vi "test-VAttributes-Merge2.vi"(8 "error in (no error)":errorcluster, 11 "TestCase in":refnum<class "MyTestCase.lvclass">) -> (0 "error out":errorcluster, 3 "TestCase out":refnum<class "MyTestCase.lvclass">)   [LabVIEW 2019, in "MyTestCase.lvclass"]
uses:
  MyTestCase.lvclass
  <vilib>/addons/_JKI Toolkits/VI Tester/TestCase.llb/TestCase.lvclass
  C:/Program Files (x86)/National Instruments/LabVIEW 2019/vi.lib/addons/_JKI Toolkits/VI Tester/TestCase.llb/TestCase.lvclass
panel:
  out "VAttributes A after B->A 2":variant
  out "VAttributes A after B->A":variant
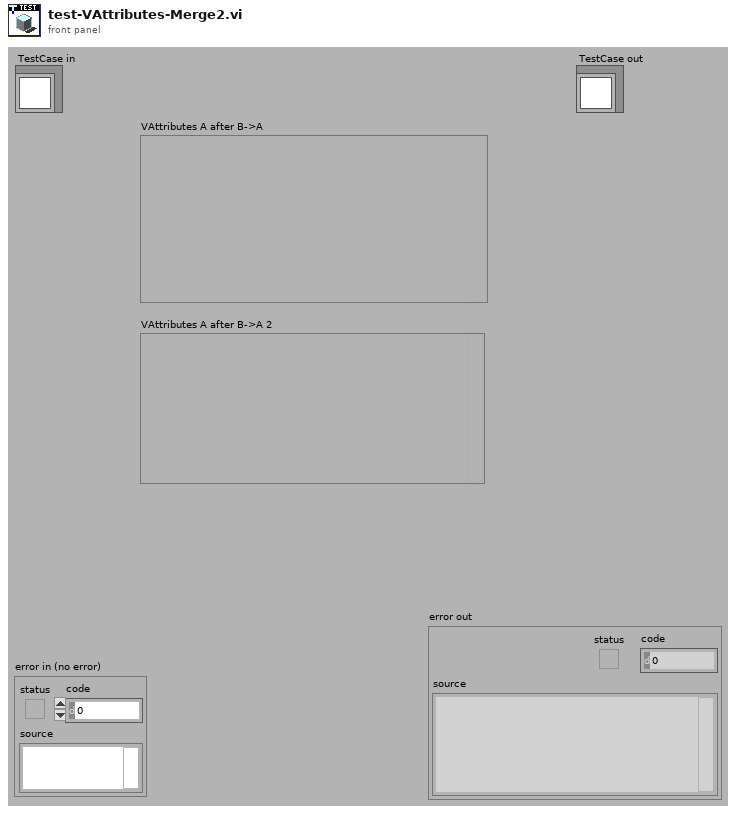
[diagram p1: front panel]
types:
  T1 = cluster{"bool":bool, "Cluster":cluster{"cluster":cluster{"cluster":cluster{"numeric":i32, "string":string}, "numeric":i32, "string":string}, "numeric":i32, "string":string}, "numeric":i32, "string":string, "string2":string}
  T2 = cluster{"numeric":i32, "string":string, "Cluster":cluster{"numeric":i32, "string":string, "cluster":cluster{"numeric":i32, "string":string, "cluster":cluster{"numeric":i32, "string":string}}}}
  T3 = cluster{"bool":bool, "string2":string, "cluster":cluster{"numeric":i32, "string":string, "cluster":cluster{"numeric":i32, "string":string}}}
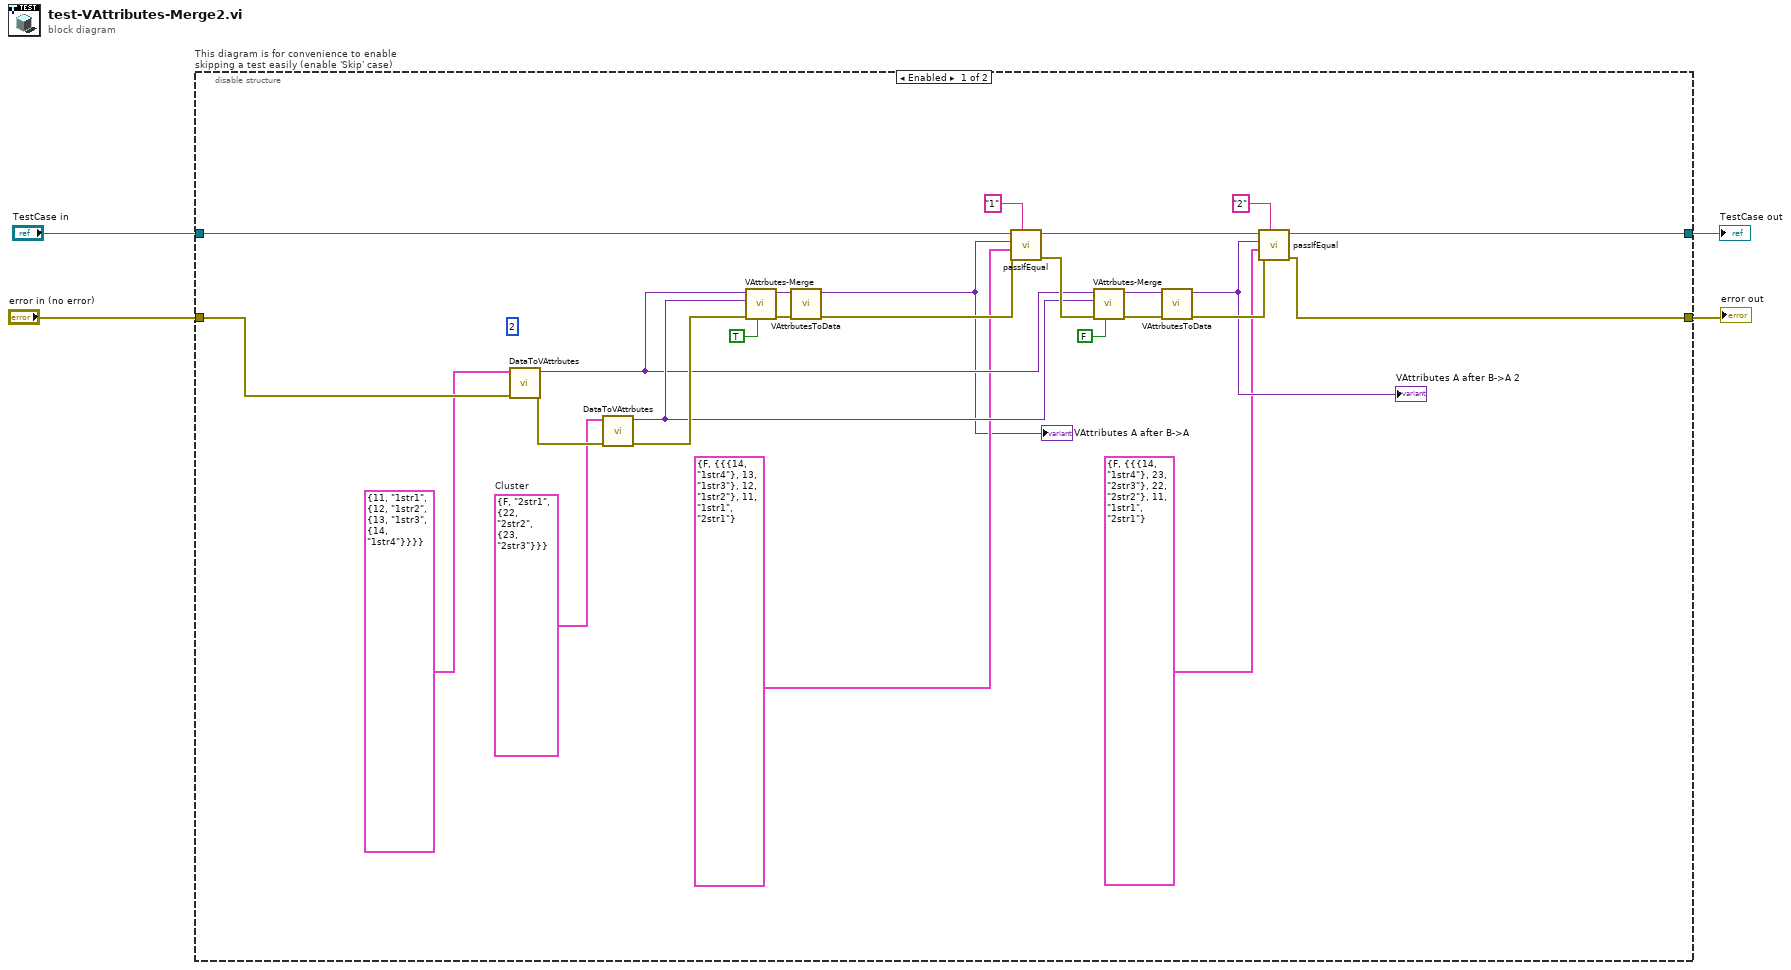
[diagram p0: block diagram]
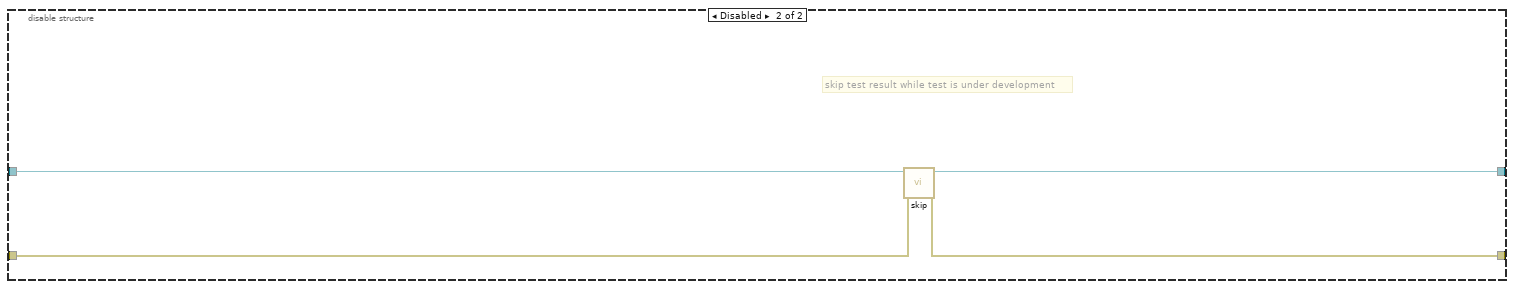
[diagram p2: hidden frame]
diagram:
  n1 = disable-structure "This diagram is for convenience to enable skipping a test easily (enable 'Skip' case)" shown="Enabled" {
    disable-tunnel: "TestCase in" -> [w27 w34]
    disable-tunnel: [w20 w32] -> w1
    disable-tunnel: [w18 w33] -> w3
    disable-tunnel: "error in (no error)" -> [w28 w31]
    frame Enabled {
      w16 = T3 {"bool"=FALSE, "string2"="2str1", "cluster"={"numeric"=22, "string"="2str2", "cluster"={"numeric"=23, "string"="2str3"}}}  # Cluster
      (unwired) 2
      n2 = call "DataToVAttrbutes.vi"("error in (no error)"=w28, "data"=T2 {"numeric"=11, "string"="1str1", "Cluster"={"numeric"=12, "string"="1str2", "cluster"={"numeric"=13, "string"="1str3", "cluster"={"numeric"=14, "string"="1str4"}}}} ("Cluster")) -> ("error out"=w30:errorcluster, "VAttributes"=w19:variant)  [unwired: 8 in]
      n3 = call "DataToVAttrbutes.vi"("error in (no error)"=w30, "data"=w16) -> ("error out"=w29:errorcluster, "VAttributes"=w21:variant)  [unwired: 8 in]
      n4 = call "VAttrbutes-Merge.vi"("If exist? Skip(T)/Overwrite(F)"=TRUE, "error in (no error)"=w29, "VAttributes B"=w21, "VAttributes A"=w19) -> ("error out"=w15:errorcluster, "VAttributes A after B->A"=w26:variant)  [unwired: 6 in]
      n5 = call "VAttrbutesToData.vi"("error in (no error)"=w15, "VAttributes"=w26) -> ("error out"=w14:errorcluster, "data"=w5:variant)  [unwired: 8 in]
      "VAttributes A after B->A" <- w5
      n6 = call-dynamic "passIfEqual.vi"("custom report message (\"\")"="1" ("custom report message (\"\")"), "error in (no error)"=w14, "y"=T1 {"bool"=FALSE, "Cluster"={"cluster"={"cluster"={"numeric"=14, "string"="1str4"}, "numeric"=13, "string"="1str3"}, "numeric"=12, "string"="1str2"}, "numeric"=11, "string"="1str1", "string2"="2str1"} ("Cluster"), "x"=w5, "TestCase in"=w27) -> ("error out"=w23:errorcluster, "TestCase out"=w22:refnum<class "MyTestCase.lvclass">)  [unwired: 5 in]
      n7 = call "VAttrbutes-Merge.vi"("If exist? Skip(T)/Overwrite(F)"=FALSE, "error in (no error)"=w23, "VAttributes B"=w21, "VAttributes A"=w19) -> ("error out"=w10:errorcluster, "VAttributes A after B->A"=w11:variant)  [unwired: 6 in]
      n8 = call "VAttrbutesToData.vi"("error in (no error)"=w10, "VAttributes"=w11) -> ("error out"=w9:errorcluster, "data"=w8:variant)  [unwired: 8 in]
      "VAttributes A after B->A 2" <- w8
      n9 = call-dynamic "passIfEqual.vi"("custom report message (\"\")"="2" ("custom report message (\"\")"), "error in (no error)"=w9, "y"=T1 {"bool"=FALSE, "Cluster"={"cluster"={"cluster"={"numeric"=14, "string"="1str4"}, "numeric"=23, "string"="2str3"}, "numeric"=22, "string"="2str2"}, "numeric"=11, "string"="1str1", "string2"="2str1"} ("Cluster"), "x"=w8, "TestCase in"=w22) -> ("error out"=w18:errorcluster, "TestCase out"=w20:refnum<class "MyTestCase.lvclass">)  [unwired: 5 in]
    }
    frame Disabled {
      # "skip test result while test is under development"
      n10 = call <vilib>:"skip.vi"("error in (no error)"=w31, "TestCase in"=w34) -> ("error out"=w33:errorcluster, "TestCase out"=w32:refnum<class "MyTestCase.lvclass">)  [unwired: 8 in]
    }
  }
  "error out" <- w3
  "TestCase out" <- w1
